vi "Go to Guiding.vi"(8 "error in (no error)":errorcluster, 11 "Guiding in":refnum<class "Guiding.lvclass">) -> (0 "error out":errorcluster, 3 "Process State out":refnum<class "State Actor.lvclass">)   [LabVIEW 2014, in "States.lvlib" / "Guiding.lvclass"]
doc: "This override disables the entry behavior when transitioning to the Running state."
uses:
  Guiding.lvclass
  <vilib>/NI/Actors/State Actor/State Actor/State Actor.lvclass
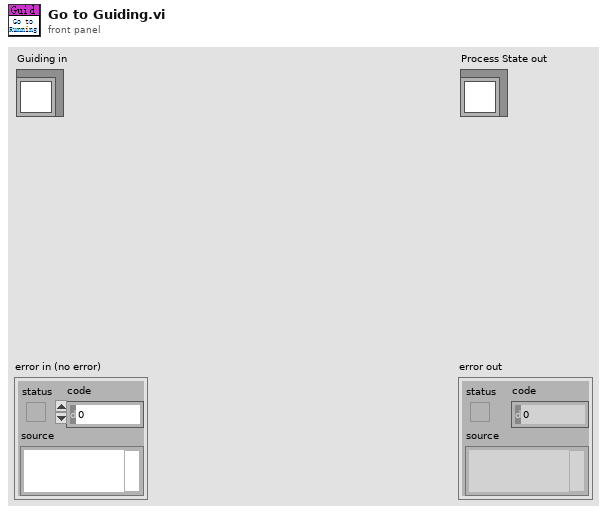
[diagram p1: front panel]
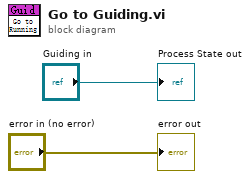
[diagram p0: block diagram]
diagram:
  "error out" <- "error in (no error)"
  "Process State out" <- "Guiding in"
